vi "Write ROI Ext.vi"(8 "error in (no error)":errorcluster, 9 "Save to File":bool=TRUE, 10 "ROI Descriptor":T1 {"Contours"."Type" items=["No Selection", "Point", "Line", "Rectangle", "Oval", "Polygon", "Freehand Region", "Annulus", "Unused2", "Unused3", "Broken Line", "Freehand Line", "Rotated Rectangle"]}, 11 "IMAQ Display in":refnum<class "HIJ Vision Display.lvclass">) -> (0 "error out":errorcluster, 3 "IMAQ Display out":refnum<class "HIJ Vision Display.lvclass">)   [LabVIEW 2020, in "HIJ Vision Display.lvlib" / "HIJ Vision Display.lvclass"]
uses:
  HIJ Vision Display.lvclass
  C:/Program Files (x86)/National Instruments/LabVIEW 2020/vi.lib/ActorFramework/Actor/Actor.lvclass
  Analyze/Analyze Parameter/Analyze Parameter ROI/Analyze Parameter ROI.lvclass
  C:/Users/AlexK/work/LabVIEW Programme/POLARIS-AS-3-Cams/Submodules/HIJ Vision/Analyze/Analyze Parameter/Analyze Parameter Base/Analyze Parameter Base.lvclass
  <vilib>/ActorFramework/Actor/Actor.lvclass/Actor.ctl
  Analyze/Analyze Parameter/Analyze Parameter ROI/Analyze Parameter ROI.lvclass/Analyze Parameter ROI.ctl
  HIJ Vision Display.lvclass/HIJ Vision Display.ctl
  Application Base Actors/HIJ Vision Application/HIJ Vision Application Messages/Set Parameter Msg/Set Parameter Msg.lvclass/Set Parameter Msg.ctl
  <vilib>/ActorFramework/Message Enqueuer/Message Enqueuer.lvclass/Message Enqueuer.ctl
  Analyze/Analyze Parameter/Analyze Parameter ROI/Write ROI Descriptor.vi
  <vilib>/ActorFramework/Message Enqueuer/Enqueue.vi
  Application Base Actors/HIJ Vision Application/HIJ Vision Application Messages/Set Parameter Msg/Set Parameter Msg.lvclass
  C:/Program Files (x86)/National Instruments/LabVIEW 2020/vi.lib/ActorFramework/Message/Message.lvclass
  <vilib>/ActorFramework/Message Priority Queue/Priority Enqueue.vi
  <vilib>/ActorFramework/Actor/Actor.lvclass
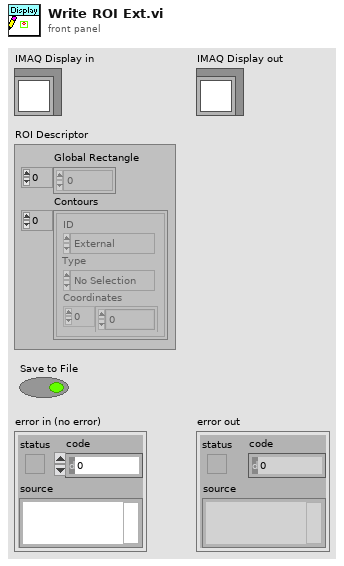
[diagram p1: front panel]
types:
  T1 = typedef "ROI Descriptor" = cluster{"Global Rectangle":i32[], "Contours":cluster{"ID":enum32{"External", "Internal"}, "Type":u32, "Coordinates":i32[]}[]}
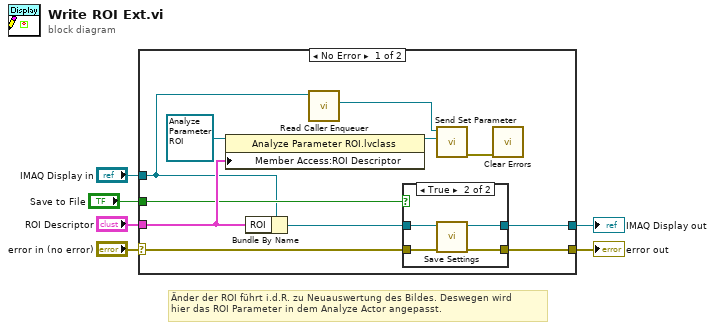
[diagram p0: block diagram]
diagram:
  # "Änder der ROI führt i.d.R. zu Neuauswertung des Bildes. Deswegen wird\nhier das ROI Parameter in dem Analyze Actor angepasst."
  n1 = case shown="No Error" "error in (no error)" {
    selector: "error in (no error)" -> [w14 w24]
    tunnel: [w13 w24] -> w5
    tunnel: [w15 w25] -> w3
    tunnel: "IMAQ Display in" -> [w7 w25]
    tunnel: "ROI Descriptor" -> [w17 _]
    tunnel: "Save to File" -> [w8 _]
    frame No Error {
      n2 = property class="Analyze Parameter ROI.lvclass"(reference=refnum<class "Analyze Parameter ROI.lvclass"> refnum ("Analyze Parameter ROI.lvclass"), "Member Access:ROI Descriptor"=w17) -> (reference out=w10:refnum<class "Analyze Parameter ROI.lvclass">)  [unwired: 1 in, 1 out]
      n3 = Bundle By Name(cluster=w7, "ROI"=w17) -> (w16:refnum<class "HIJ Vision Display.lvclass">)
      n4 = call <vilib>:"Read Caller Enqueuer.vi"("Actor"=w7) -> ("Caller Enqueuer"=w11:refnum<class "Message Enqueuer.lvclass">)  [unwired: 10 in]
      n5 = case shown="True" w8 {
        tunnel: w16 -> [w19 w23]
        tunnel: [w19 w22] -> w15
        tunnel: w14 -> [w18 w21]
        tunnel: [w18 w20] -> w13
        frame False {
        }
        frame True {
          n6 = call-dynamic "Save Settings.vi"("error in (no error)"=w21, "IMAQ Display in"=w23) -> ("error out"=w20:errorcluster, "IMAQ Display out"=w22:refnum<class "HIJ Vision Display.lvclass">)  [unwired: 8 in]
        }
      }
      n7 = call "Send Set Parameter.vi"("Parameter"=w10, "Message Enqueuer"=w11) -> ("error out"=w9:errorcluster)  [unwired: 8 in, 1 out]
      n8 = call <vilib>:"Clear Errors.vi"("error in (no error)"=w9) -> ()  [unwired: 5 in, 2 out]
    }
    frame Error {
    }
  }
  "error out" <- w5
  "IMAQ Display out" <- w3
